vi "ENAinit.vi"(2 "Error In (no error)":errorcluster, 3 "Meas":T2, 4 "ENA Config":T1={"Sweep Type"=0, "Sweep Mode"=0, "Sweep Points"=201, "Average count"=16, "IF Bandwidth (Hz)"=100000.0, "Power Level (dBm)"=0.0, "Center Freq (Hz)"=0.0, "Span Freq (Hz)"=0.0, "Electrical Delay (s)"=0.0} {"Electrical Delay (s)" format="%.2p"; "Span Freq (Hz)" format="%.2p"; "Center Freq (Hz)" format="%.2p"; "Power Level (dBm)" format="%^.2g"; "IF Bandwidth (Hz)" format="%.1p"; "Sweep Mode" items=["Stepped", "Swept", "Fast Stepped Mode", "Fast Swept Mode"]; "Sweep Type" items=["Linear Sweep", "Logarithmic Sweep", "Segment Sweep", "Power Sweep", "DC Bias"]}, 5 "VISA session":refnum<visa-resource-name>) -> (0 "Error Out":errorcluster, 1 "dup VISA session":refnum<visa-resource-name>)   [LabVIEW 2017]
uses:
  <instrlib>/Agilent ENA Series/Agilent ENA Series.lvlib
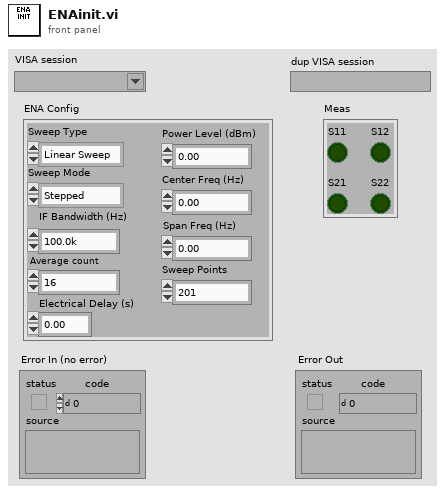
[diagram p1: front panel]
types:
  T1 = cluster{"Sweep Type":u16, "Sweep Mode":u16, "Sweep Points":i32, "Average count":i32, "IF Bandwidth (Hz)":dbl, "Power Level (dBm)":dbl, "Center Freq (Hz)":dbl, "Span Freq (Hz)":dbl, "Electrical Delay (s)":dbl}
  T2 = cluster{"S11":bool, "S12":bool, "S21":bool, "S22":bool}
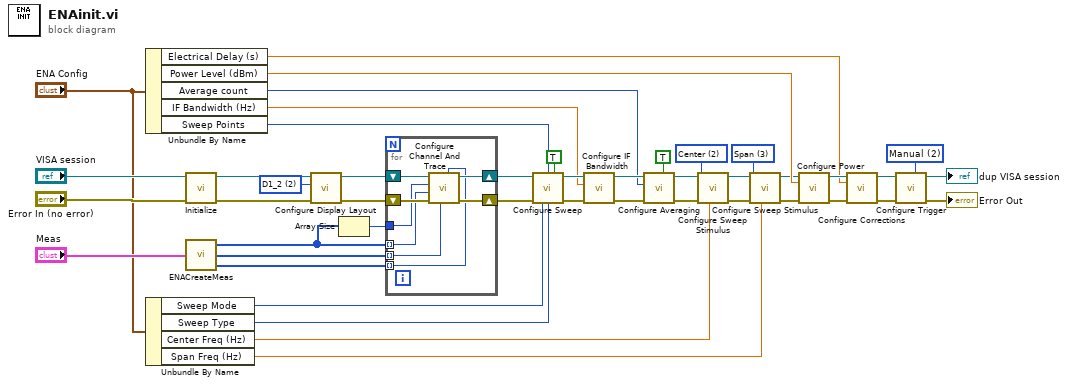
[diagram p0: block diagram]
diagram:
  w1 = u16 2 items=["Internal", "External", "Manual", "BUS"] ("Trigger Source (0: Internal)")
  w14 = u16 2 items=["D1", "D12", "D1_2", "D112", "D1_1_2", "D123", "D1_2_3", "D12_33", "D11_23", "D13_23", "D12_13", "D1234", "D1_2_3_4", "D12_34", "D123_456", "D12_34_56", "D1234_5678", "D12_34_56_78", "D123_456_789", "D123_ABC", "D1234_9ABC", "D123_CDEF"] ("Graph Layout (0:D1)")
  w24 = u16 3 items=["Start", "Stop", "Center", "Span"] ("Stimulus (0: Start)")
  w25 = u16 2 items=["Start", "Stop", "Center", "Span"] ("Stimulus (0: Start)")
  n1 = Unbundle By Name("ENA Config") -> ("Electrical Delay (s)"=w31:dbl, "Power Level (dBm)"=w30:dbl, "Average count"=w35:i32, "IF Bandwidth (Hz)"=w41:dbl, "Sweep Points"=w20:i32)
  n2 = Unbundle By Name("ENA Config") -> ("Sweep Mode"=w18:u16, "Sweep Type"=w19:u16, "Center Freq (Hz)"=w23:dbl, "Span Freq (Hz)"=w22:dbl)
  n3 = call <instrlib>:"Initialize.vi"("error in (no error)"="Error In (no error)", "VISA resource name"="VISA session") -> ("error out"=w15:errorcluster, "VISA resource name out"=w16:refnum<visa-resource-name>)  [unwired: 8 in]
  n4 = call "ENACreateMeas.vi"("Meas in"="Meas") -> ("Meas parameters"=w11:u16[], "Data format"=w13:u16[], "Active trace"=w12:i32[])
  n5 = call <instrlib>:"Configure Display Layout.vi"("error in (no error)"=w15, "Graph Layout (0:D1)"=w14, "VISA resource name"=w16) -> ("error out"=w8:errorcluster, "VISA resource name out"=w9:refnum<visa-resource-name>)  [unwired: 7 in]
  n6 = Array Size(array=w11) -> (size(s)=w10:i32)
  n7 = for {
    tunnel: w11 -> [w48] mode=indexing
    tunnel: w13 -> [w47] mode=indexing
    tunnel: w12 -> [w46] mode=indexing
    tunnel: w10 -> [w49]
    shift-right: [w52] -> w7
    shift-left: w9 -> [w53]
    shift-right: [w50] -> w6
    shift-left: w8 -> [w51]
    n8 = call <instrlib>:"Configure Channel And Trace.vi"("Active Trace (1)"=w46, "Data Format (0: Logarithmic Magnitude)"=w47, "error in (no error)"=w51, "Measurement Parameters (0: S11)"=w48, "Number of Traces (1)"=w49, "VISA resource name"=w53) -> ("error out"=w50:errorcluster, "VISA resource name out"=w52:refnum<visa-resource-name>)  [unwired: 4 in]
  }
  n9 = call <instrlib>:"Configure Sweep.vi"("VISA resource name"=w7, "Number of Measurement Points (201)"=w20, "Auto Sweep Time (F: Off)"=TRUE ("Sweep Time Auto"), "error in (no error)"=w6, "Sweep Mode (0: Stepped)"=w18, "Sweep Type (0: Linear Sweep)"=w19) -> ("VISA resource name out"=w44:refnum<visa-resource-name>, "error out"=w43:errorcluster)  [unwired: 8 in]
  n10 = call <instrlib>:"Configure IF Bandwidth.vi"("error in (no error)"=w43, "IF Bandwidth (100000.0)"=w41, "VISA resource name"=w44) -> ("error out"=w39:errorcluster, "VISA resource name out"=w37:refnum<visa-resource-name>)  [unwired: 7 in]
  n11 = call <instrlib>:"Configure Averaging.vi"("Averaging State (F: Off)"=TRUE ("Average State (F: Off)"), "error in (no error)"=w39, "Factor (16)"=w35, "VISA resource name"=w37) -> ("error out"=w38:errorcluster, "VISA resource name out"=w36:refnum<visa-resource-name>)  [unwired: 6 in]
  n12 = call <instrlib>:"Configure Sweep Stimulus.vi"("Parameter (0.0)"=w23, "error in (no error)"=w38, "Stimulus (0: Start)"=w25, "VISA resource name"=w36) -> ("error out"=w26:errorcluster, "VISA resource name out"=w29:refnum<visa-resource-name>)  [unwired: 6 in]
  n13 = call <instrlib>:"Configure Sweep Stimulus.vi"("Parameter (0.0)"=w22, "error in (no error)"=w26, "Stimulus (0: Start)"=w24, "VISA resource name"=w29) -> ("error out"=w27:errorcluster, "VISA resource name out"=w28:refnum<visa-resource-name>)  [unwired: 6 in]
  n14 = call <instrlib>:"Configure Power.vi"("VISA resource name"=w28, "Power Level (0.0)"=w30, "error in (no error)"=w27) -> ("VISA resource name out"=w33:refnum<visa-resource-name>, "error out"=w32:errorcluster)  [unwired: 11 in]
  n15 = call <instrlib>:"Configure Corrections.vi"("VISA resource name"=w33, "Electrical DelayTime (0.0)"=w31, "error in (no error)"=w32) -> ("VISA resource name out"=w5:refnum<visa-resource-name>, "error out"=w4:errorcluster)  [unwired: 11 in]
  n16 = call <instrlib>:"Configure Trigger.vi"("Trigger Source (0: Internal)"=w1, "error in (no error)"=w4, "VISA resource name"=w5) -> ("error out"=→"Error Out":errorcluster, "VISA resource name out"=→"dup VISA session":refnum<visa-resource-name>)  [unwired: 7 in]
